vi "test1-AllWOrkerNodesShareTheSameData.vi"(8 "error in (no error)":errorcluster, 11 "TestCase in":refnum<class "testcase-CSMWorkerMode.lvclass">) -> (0 "error out":errorcluster, 3 "TestCase out":refnum<class "testcase-CSMWorkerMode.lvclass">)   [LabVIEW 2017, in "testcase-CSMWorkerMode.lvclass"]
uses:
  testcase-CSMWorkerMode.lvclass
  src/user.lib/_NEVSTOP/Communicable State Machine(CSM)/_Support/Typedef/_CSM_MODE.ctl
  9c2ff45f-acc9-407c-894c-164613e63933.vi
  <vilib>/addons/_JKI Toolkits/VI Tester/TestCase.llb/TestCase.lvclass
  src/user.lib/_NEVSTOP/Communicable State Machine(CSM)/Communicable State Machine.lvlib
  C:/Program Files (x86)/National Instruments/LabVIEW 2017/vi.lib/addons/_JKI Toolkits/VI Tester/TestCase.llb/TestCase.lvclass
panel:
  out "LoopCount":i32
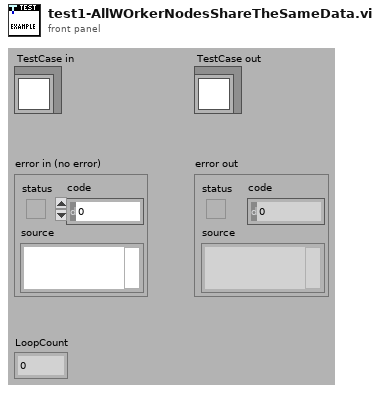
[diagram p1: front panel]
types:
  T1 = typedef "Communicable State Machine.lvlib/_CSM_MODE.ctl" = enum16{"Not Exist", "Stand Alone", "CSM", "Worker", "Worker Agent", "Chain Node", "Chain"}
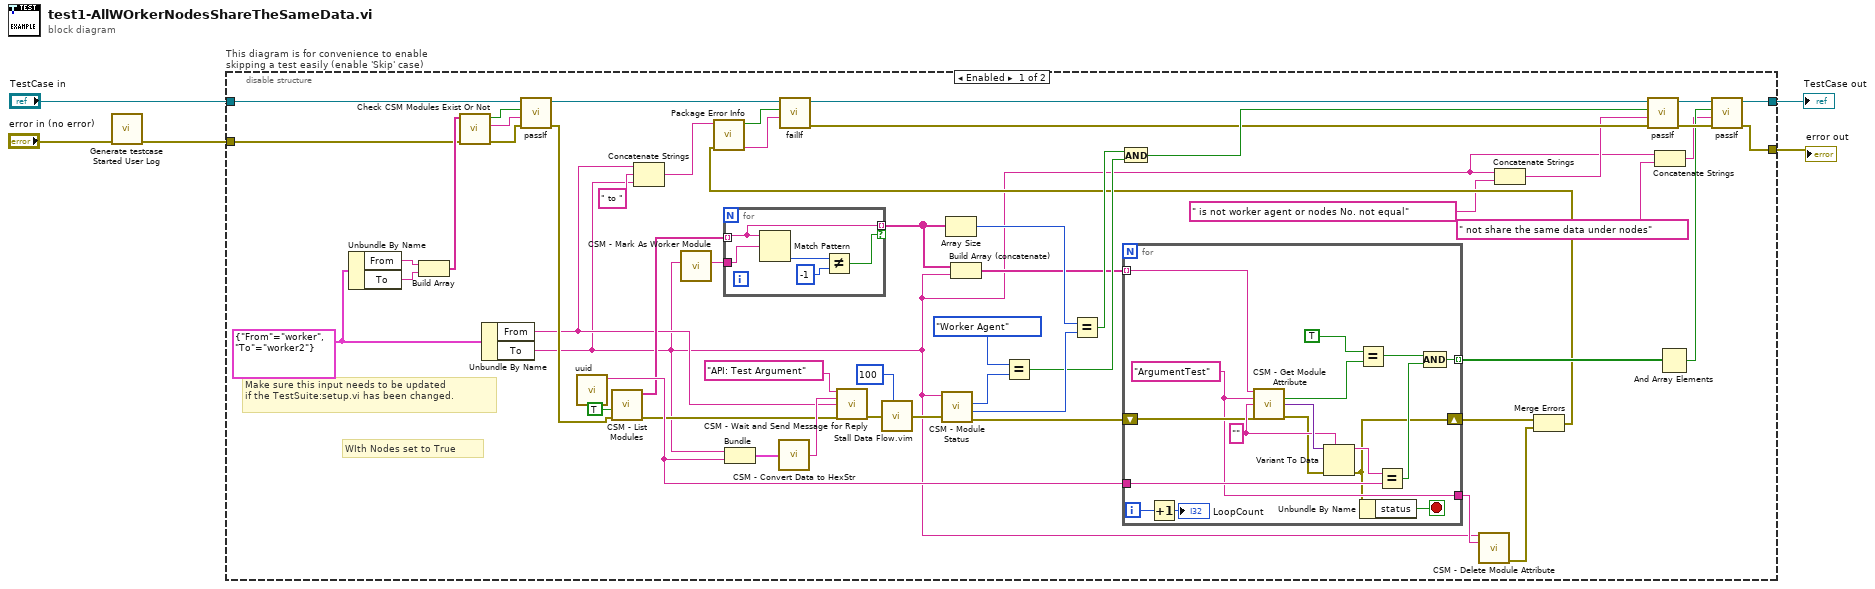
[diagram p0: block diagram]
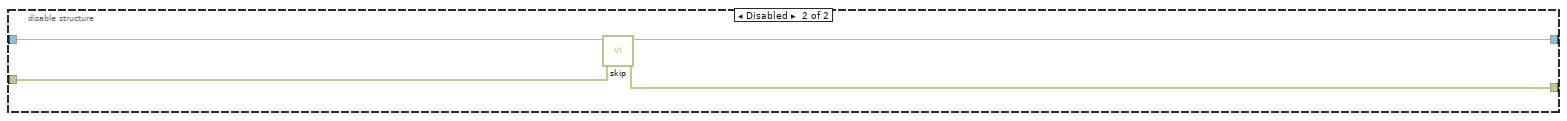
[diagram p2: hidden frame]
diagram:
  n1 = call "Generate testcase Started User Log.vi"("Error In"="error in (no error)") -> ("error out"=w1:errorcluster)  [unwired: 10 in]
  n2 = disable-structure "This diagram is for convenience to enable skipping a test easily (enable 'Skip' case)" shown="Enabled" {
    disable-tunnel: "TestCase in" -> [w19 w85]
    disable-tunnel: [w40 w83] -> w2
    disable-tunnel: [w38 w84] -> w4
    disable-tunnel: w1 -> [w20 w82]
    frame Enabled {
      w27 = cluster{"From":string, "To":string} {"From"="worker", "To"="worker2"} ("Cluster")
      # "Make sure this input needs to be updated \nif the TestSuite:setup.vi has been changed."
      # "WIth Nodes set to True"
      n3 = Unbundle By Name(w27) -> ("From"=w22:string, "To"=w23:string)
      n4 = Build Array(w22, w23) -> (w21:string[])
      n5 = call "Check CSM Modules Exist Or Not.vi"("error in"=w20, "CSM names in"=w21) -> ("error out"=w24:errorcluster, "Debug string"=w25:string, "All Modules Exist?"=w26:bool)  [unwired: 7 in]
      n6 = Unbundle By Name(w27) -> ("From"=w16:string, "To"=w8:string)
      n7 = call-dynamic "passIf.vi"("error in (no error)"=w24, "message (\"\")"=w25, "pass"=w26, "TestCase in"=w19) -> ("error out"=w18:errorcluster, "TestCase out"=w13:refnum<class "testcase-CSMWorkerMode.lvclass">)  [unwired: 6 in]
      n8 = call "uuid.vi"() -> ("UUID"=w54:string)  [unwired: 11 in]
      n9 = call "CSM - List Modules.vi"("Error In"=w18, "With Nodes? (F)"=TRUE) -> ("error out"=w48:errorcluster, "Module Names"=w51:string[])  [unwired: 8 in]
      n10 = Concatenate Strings(w16, " to " ("string"), w8) -> (w14:string)
      n11 = call "CSM - Mark As Worker Module.vi"("CSM Name"=w8) -> ("CSM Name (Marked As Worker)"=w47:string)  [unwired: 9 in]
      n12 = for {
        tunnel: w51 -> [w79] mode=indexing
        tunnel: [w79] -> w37 mode=indexing if=w78
        tunnel: w47 -> [w77]
        n13 = Match Pattern(string=w79, regular expression=w77) -> (offset past match=w81:i32)  [unwired: 1 in, 3 out]
        n14 = Not Equal?(x=w81, y=-1) -> (x != y?=w78:bool)
      }
      n15 = Bundle("To"=w8, "UUID"=w54) -> (w56:cluster{"To":string, "UUID":string})  [unwired: 1 in]
      n16 = call "CSM - Convert Data to HexStr.vi"("Variant"=w56) -> ("HEX String (0-9,A-F)"=w55:string)  [unwired: 8 in]
      n17 = call "CSM - Wait and Send Message for Reply.vi"("State"="API: Test Argument", "Arguments (\"\")"=w55, "Target Module"=w16, "Error In (No Error)"=w48) -> ("error out"=w58:errorcluster)  [unwired: 8 in, 3 out]
      n18 = call "Stall Data Flow.vim"("value in"=w58, "milliseconds to wait"=u32 100) -> ("value out"=w53:errorcluster)  [unwired: 1 out]
      n19 = call "CSM - Module Status.vi"("Error In"=w53, "CSM Name"=w8) -> ("error out"=w35:errorcluster, "#Nodes"=w46:i32, "Mode"=w49:T1)  [unwired: 5 in, 2 out]
      n20 = Array Size(array=w37) -> (size(s)=w45:i32)
      n21 = Build Array (concatenate)(w37, w8) -> (w36:string[])
      n22 = Equal?(x=_CSM_MODE."Worker Agent" ("Mode 2"), y=w49) -> (x = y?=w43:bool)
      n23 = Equal?(x=w45, y=w46) -> (x = y?=w44:bool)
      n24 = And(x=w44, y=w43) -> (x .and. y?=w42:bool)
      n25 = for {
        tunnel: w54 -> [w76]
        tunnel: w36 -> [w67] mode=indexing
        shift-right: [w61] -> w31
        shift-left: w35 -> [w66]
        tunnel: [w65] -> w34 mode=indexing
        tunnel: [w64] -> w32
        i -> [w63]
        stop <- w60 stop-if-true
        w72 = ""
        w64 = "ArgumentTest" ("Attribute")
        n26 = Increment(x=w63) -> (x+1=→"LoopCount":i32)
        n27 = call "CSM - Get Module Attribute.vi"("CSM Name"=w67, "Attribute"=w64, "Default Value (Empty Variant)"=w72, "Error In"=w66) -> ("Found"=w75:bool, "Value"=w73:variant, "error out"=w70:errorcluster)  [unwired: 7 in, 2 out]
        n28 = Variant To Data(error in=w70, type=w72, Variant=w73) -> (data=w71:string, error out=w61:errorcluster)
        n29 = Equal?(x=TRUE, y=w75) -> (x = y?=w69:bool)
        n30 = Unbundle By Name(w61) -> ("status"=w60:bool)
        n31 = Equal?(x=w71, y=w76) -> (x = y?=w68:bool)
        n32 = Compound Arithmetic op=AND(w69, w68) -> (w65:bool)
      }
      n33 = call "CSM - Delete Module Attribute.vi"("CSM Name"=w8, "Attribute"=w32) -> ("error out"=w30:errorcluster)  [unwired: 10 in, 3 out]
      n34 = Concatenate Strings(w8, " is not worker agent or nodes No. not equal" ("string")) -> (w10:string)
      n35 = Merge Errors(w31, w30) -> (w17:errorcluster)
      n36 = call "Package Error Info.vi"("error in"=w17, "String in"=w14) -> ("packed error info out"=w28:string, "error status"=w29:bool)  [unwired: 8 in]
      n37 = call-dynamic "failIf.vi"("message (\"\")"=w28, "fail"=w29, "TestCase in"=w13) -> ("error out"=w12:errorcluster, "TestCase out"=w11:refnum<class "testcase-CSMWorkerMode.lvclass">)  [unwired: 7 in]
      n38 = call-dynamic "passIf.vi"("error in (no error)"=w12, "message (\"\")"=w10, "pass"=w42, "TestCase in"=w11) -> ("error out"=w39:errorcluster, "TestCase out"=w41:refnum<class "testcase-CSMWorkerMode.lvclass">)  [unwired: 6 in]
      n39 = Concatenate Strings(w8, " not share the same data under nodes" ("string")) -> (w6:string)
      n40 = And Array Elements(Boolean array=w34) -> (logical AND=w33:bool)
      n41 = call-dynamic "passIf.vi"("error in (no error)"=w39, "message (\"\")"=w6, "pass"=w33, "TestCase in"=w41) -> ("error out"=w38:errorcluster, "TestCase out"=w40:refnum<class "testcase-CSMWorkerMode.lvclass">)  [unwired: 6 in]
    }
    frame Disabled {
      # "skip test result while test is under development"
      n42 = call <vilib>:"skip.vi"("error in (no error)"=w82, "TestCase in"=w85) -> ("error out"=w84:errorcluster, "TestCase out"=w83:refnum<class "testcase-CSMWorkerMode.lvclass">)  [unwired: 8 in]
    }
  }
  "error out" <- w4
  "TestCase out" <- w2
